vi "OSICS_Get_Power.vi"(7 "OSICS slot":i32=1 min=1 max=8 step=1, 8 "error in":errorcluster, 10 "Power Unit(False: dBm)":bool, 11 "VISA IN":refnum<visa-resource-name>) -> (0 "error out":errorcluster, 1 "Laser State (False:Disabled)":bool, 2 "Power (dBm/mW)":dbl format="%.2f", 3 "VISA OUT":refnum<visa-resource-name>, 5 "ERR":i32)   [LabVIEW 2014, in "OSICS_LIB.lvlib"]
doc: "This Vi reads the power settings of the OSICS modules depending on the input power unit."
uses:
  OSICS_LIB.lvlib
panel:
  # "Basic Function to read the power settings\nof the OSICS"
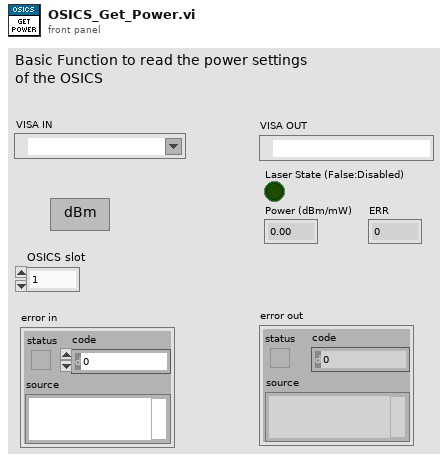
[diagram p1: front panel]
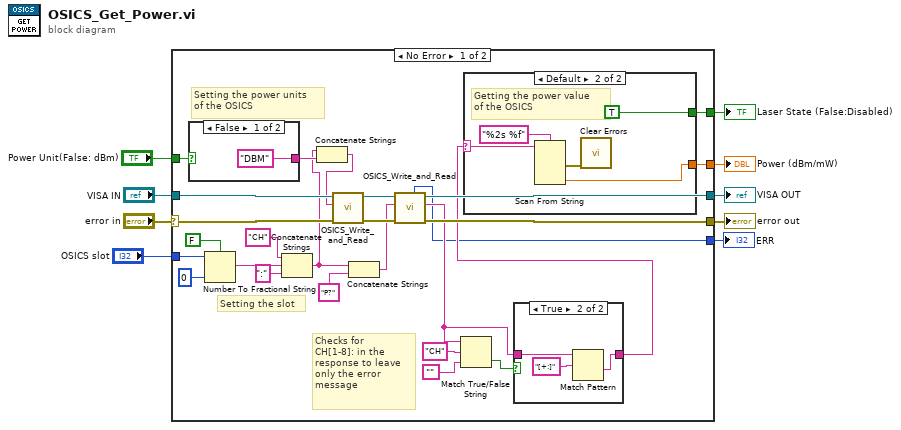
[diagram p0: block diagram]
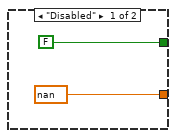
[diagram p3: hidden frame]
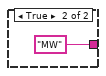
[diagram p4: hidden frame]
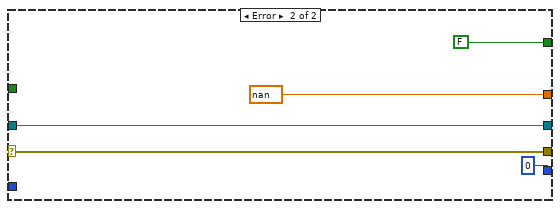
[diagram p5: hidden frame]
diagram:
  n1 = case shown="No Error" "error in" {
    selector: "error in" -> [w34 w52]
    tunnel: "Power Unit(False: dBm)" -> [w32 _]
    tunnel: "VISA IN" -> [w35 w53]
    tunnel: [w31 w53] -> w8
    tunnel: [w30 w52] -> w7
    tunnel: [w33 nan] -> w5
    tunnel: [w27 FALSE] -> w3
    tunnel: [w10 0 ("ERR")] -> w2
    tunnel: "OSICS slot" -> [w26 _]
    frame No Error {
      # "Checks for \nCH[1-8]: in the\nresponse to leave\nonly the error\nmessage"
      # "Setting the slot"
      # "Setting the power units\nof the OSICS"
      n2 = case shown="False" w32 {
        tunnel: ["DBM" "MW"] -> w20
        frame False {
        }
        frame True {
        }
      }
      n3 = Number To Fractional String(use system decimal point (T)=FALSE, number=w26, precision (6)=i16 0) -> (F-format string=w22:string)  [unwired: 1 in]
      n4 = Concatenate Strings("CH" ("string"), w22, ":" ("string")) -> (w18:string)
      n5 = Concatenate Strings(w18, w20) -> (w19:string)
      n6 = call "OSICS_Write_and_Read.vi"("error in (no error)"=w34, "String to Send"=w19, "VISA IN"=w35) -> ("error out"=w28:errorcluster, "VISA OUT"=w29:refnum<visa-resource-name>)  [unwired: 5 in, 2 out]
      n7 = Concatenate Strings(w18, "P?" ("string")) -> (w16:string)
      n8 = call "OSICS_Write_and_Read.vi"("error in (no error)"=w28, "String to Send"=w16, "VISA IN"=w29) -> ("error out"=w30:errorcluster, "Message Available"=w12:string, "VISA OUT"=w31:refnum<visa-resource-name>, "ERR"=w10:i32)  [unwired: 5 in]
      n9 = Match True/False String(2:"", 3:"CH" ("true string"), 4:w12) -> (0:w13:bool)  [unwired: 1 out]
      n10 = case shown="True" w13 {
        tunnel: w12 -> [w36 w38]
        tunnel: [w36 w37] -> w11
        frame False {
        }
        frame True {
          n11 = Match Pattern(string=w38, regular expression="[+:]") -> (after substring=w37:string)  [unwired: 1 in, 3 out]
        }
      }
      n12 = case shown="Default" w11 {
        selector: w11 -> [_ w44]
        tunnel: [nan w45] -> w33
        tunnel: [FALSE TRUE] -> w27
        frame "Disabled" {
        }
        frame Default {
          # "Getting the power value\nof the OSICS"
          n13 = Scan From String(format string="%2s %f", input string=w44) -> (error out=w42:errorcluster, output 2=w45:dbl)  [unwired: 5 in, 2 out]
          n14 = call <vilib>:"Clear Errors.vi"("error in (no error)"=w42) -> ()  [unwired: 5 in, 2 out]
        }
      }
    }
    frame Error {
    }
  }
  "error out" <- w7
  "VISA OUT" <- w8
  "Power (dBm/mW)" <- w5
  "Laser State (False:Disabled)" <- w3
  "ERR" <- w2
